vi "LX-ShowP_F_R.vi"(0 "ng/ok":bool) -> (4 "TotaNumber":string, 6 "PassNumber":string, 8 "FailNumber":string, 10 "fail 个数":i32, 15 "Pass 个数":i32)   [LabVIEW 2017]
uses:
  Global System.vi
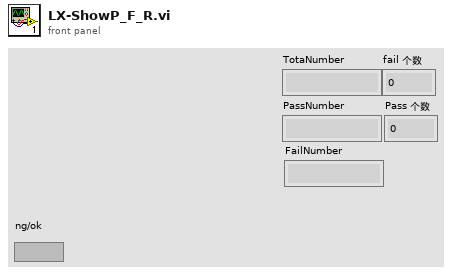
[diagram p1: front panel]
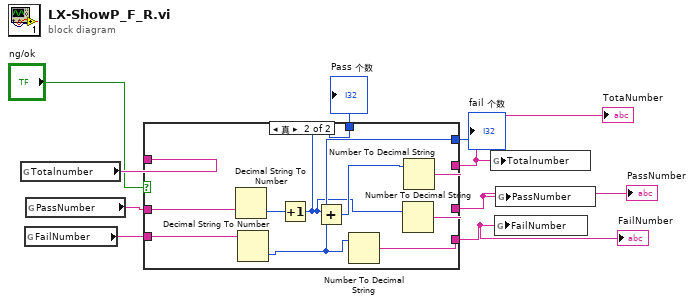
[diagram p0: block diagram]
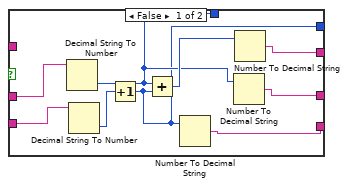
[diagram p2: hidden frame]
diagram:
  n1 = global read "Global System.vi" "Totalnumber"() -> (w9:string)
  n2 = global read "Global System.vi" "FailNumber"() -> (w7:string)
  n3 = global read "Global System.vi" "PassNumber"() -> (w8:string)
  n4 = case shown="真" "ng/ok" {
    tunnel: w9 -> [_ _]
    tunnel: w8 -> [w17 w27]
    tunnel: w7 -> [w16 w26]
    tunnel: [w15 w23] -> w6
    tunnel: [w14 w22] -> w4
    tunnel: [w13 w21] -> w3
    tunnel: [w12 w19] -> w1
    tunnel: [w10 w20] -> w2
    frame False {
      n5 = Decimal String To Number(string=w17) -> (number=w12:i32)  [unwired: 2 in, 1 out]
      n6 = Decimal String To Number(string=w16) -> (number=w11:i32)  [unwired: 2 in, 1 out]
      n7 = Increment(x=w11) -> (x+1=w10:i32)
      n8 = Add(x=w12, y=w10) -> (x+y=w18:i32)
      n9 = Number To Decimal String(number=w10) -> (decimal integer string=w13:string)  [unwired: 1 in]
      n10 = Number To Decimal String(number=w12) -> (decimal integer string=w14:string)  [unwired: 1 in]
      n11 = Number To Decimal String(number=w18) -> (decimal integer string=w15:string)  [unwired: 1 in]
    }
    frame True {
      n12 = Decimal String To Number(string=w27) -> (number=w25:i32)  [unwired: 2 in, 1 out]
      n13 = Decimal String To Number(string=w26) -> (number=w20:i32)  [unwired: 2 in, 1 out]
      n14 = Increment(x=w25) -> (x+1=w19:i32)
      n15 = Add(x=w19, y=w20) -> (x+y=w24:i32)
      n16 = Number To Decimal String(number=w20) -> (decimal integer string=w21:string)  [unwired: 1 in]
      n17 = Number To Decimal String(number=w19) -> (decimal integer string=w22:string)  [unwired: 1 in]
      n18 = Number To Decimal String(number=w24) -> (decimal integer string=w23:string)  [unwired: 1 in]
    }
  }
  "TotaNumber" <- w6
  "PassNumber" <- w4
  "FailNumber" <- w3
  "fail 个数" <- w2
  "Pass 个数" <- w1
  n19 = global write "Global System.vi" "Totalnumber"(w6) -> ()
  n20 = global write "Global System.vi" "FailNumber"(w3) -> ()
  n21 = global write "Global System.vi" "PassNumber"(w4) -> ()
